vi "Swerve Math.vi"(9 "Yaw":dbl=-5.71, 10 "Rot. Point Y":dbl, 11 "Rot. Point X":dbl) -> (3 "Swerve Math Ouput":dbl[](array[numeric])=[0.0, 0.0, 0.0, 0.0, 0.0, 10.75, 16.677080080157918, 12.75])   [LabVIEW 2018]
uses:
  Drive Train Global.vi
  Robot Information/Robot Information Global.vi
  <vilib>/addons/control/pid/pid.llb/PID (DBL).vi
  <vilib>/addons/control/pid/NI_PID_pid.lvlib
panel:
  in  "PID gains":T1={"proportional gain (Kc)"=0.03, "integral time (Ti, min)"=0.0, "derivative time (Td, min)"=0.001} {"derivative time (Td, min)" format="%.3f"; "integral time (Ti, min)" format="%.3f"; "proportional gain (Kc)" format="%.3f"}
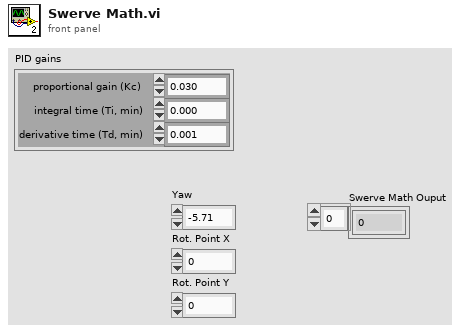
[diagram p1: front panel]
types:
  T1 = cluster{"proportional gain (Kc)":dbl, "integral time (Ti, min)":dbl, "derivative time (Td, min)":dbl}
  T2 = cluster{"Rollover":dbl, "Yaw":dbl, "Cont Yaw":dbl}
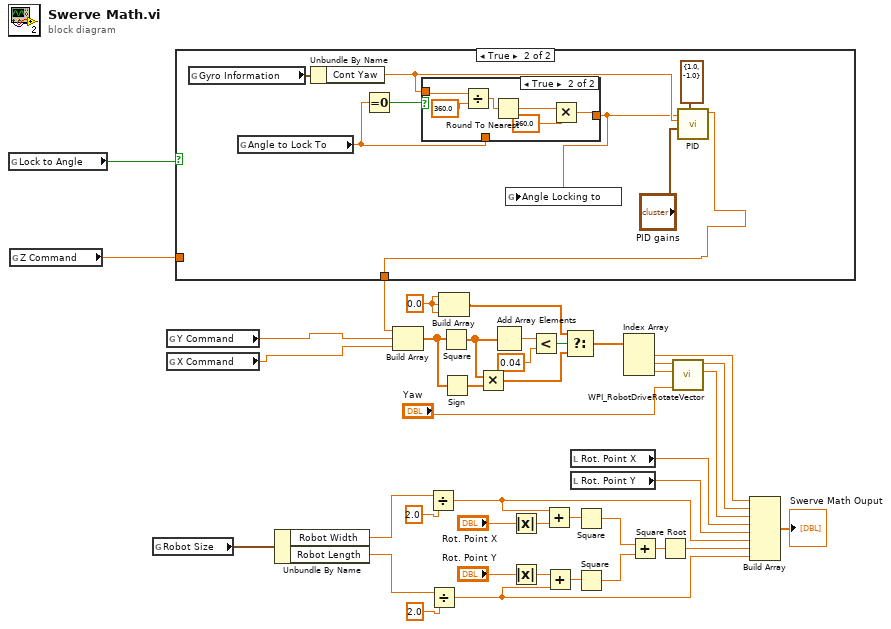
[diagram p0: block diagram]
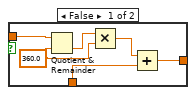
[diagram p3: hidden frame]
diagram:
  w12 = 0.0 ("element")
  n1 = global read "Drive Train Global.vi" "Lock to Angle"() -> (w4:bool)
  n2 = global read "Drive Train Global.vi" "Z Command"() -> (w5:dbl)
  n3 = global read "Robot Information Global.vi" "Robot Size"() -> (w19:cluster{"Robot Width":dbl, "Robot Length":dbl})
  n4 = global read "Drive Train Global.vi" "Y Command"() -> (w2:dbl)
  n5 = global read "Drive Train Global.vi" "X Command"() -> (w1:dbl)
  n6 = case shown="True" w4 {
    tunnel: [w42 w43] -> w3
    tunnel: w5 -> [w42 _]
    frame False {
    }
    frame True {
      n7 = global read "Drive Train Global.vi" "Gyro Information"() -> (w50:T2)
      n8 = global read "Drive Train Global.vi" "Angle to Lock To"() -> (w45:dbl)
      n9 = Unbundle By Name(w50) -> ("Cont Yaw"=w47:dbl)
      n10 = Equal To 0?(x=w45) -> (x = 0?=w44:bool)
      n11 = case shown="True" w44 {
        tunnel: w47 -> [w56 w62]
        tunnel: w45 -> [w55 _]
        tunnel: [w54 w57] -> w46
        frame False {
          w52 = 360.0 ("y")
          n12 = Quotient & Remainder(x=w56, y=w52) -> (floor(x/y)=w53:dbl)  [unwired: 1 out]
          n13 = Multiply(x=w53, y=w52) -> (x*y=w51:dbl)
          n14 = Add(x=w51, y=w55) -> (x+y=w54:dbl)
        }
        frame True {
          n15 = Divide(x=w62, y=360.0) -> (x/y=w60:dbl)
          n16 = Round To Nearest(number=w60) -> (nearest integer value=w59:dbl)
          n17 = Multiply(x=w59, y=360.0) -> (x*y=w57:dbl)
        }
      }
      n18 = global write "Drive Train Global.vi" "Angle Locking to"(w46) -> ()
      n19 = call-poly <vilib>:"PID.vi"("output range"=cluster{"output high":dbl, "output low":dbl} {"output high"=1.0, "output low"=-1.0}, "PID gains"="PID gains", "process variable"=w47, "setpoint"=w46) -> ("output"=w43:dbl)  [unwired: 6 in, 1 out]
    }
  }
  n20 = Unbundle By Name(w19) -> ("Robot Width"=w17:dbl, "Robot Length"=w18:dbl)
  n21 = Build Array(w3, w2, w1) -> (w8:dbl[])
  n22 = Divide(x=w17, y=2.0) -> (x/y=w27:dbl)
  n23 = Divide(x=w18, y=2.0) -> (x/y=w25:dbl)
  n24 = Build Array(w12, w12, w12) -> (w13:dbl[])
  n25 = Square(x=w8) -> (x^2=w10:dbl[])
  n26 = Sign(1:w8) -> (0:w11:dbl[])
  n27 = Multiply(x=w10, y=w11) -> (x*y=w9:dbl[])
  n28 = Add Array Elements(numeric array=w10) -> (sum=w16:dbl)
  n29 = Absolute Value(x="Rot. Point X") -> (abs(x)=w41:dbl)
  n30 = Absolute Value(x="Rot. Point Y") -> (abs(x)=w39:dbl)
  n31 = Less?(x=w16, y=0.04 ("x")) -> (x < y?=w14:bool)
  n32 = Add(x=w27, y=w41) -> (x+y=w40:dbl)
  n33 = Add(x=w39, y=w25) -> (x+y=w38:dbl)
  n34 = Select(t=w13, s=w14, f=w9) -> (s? t:f=w23:dbl[])
  n35 = local read "Rot. Point X"() -> (w29:dbl)
  n36 = local read "Rot. Point Y"() -> (w28:dbl)
  n37 = Square(x=w40) -> (x^2=w36:dbl)
  n38 = Square(x=w38) -> (x^2=w37:dbl)
  n39 = Index Array(array=w23) -> (element #1=w21:dbl, element #2=w24:dbl, element #3=w30:dbl)  [unwired: 3 in]
  n40 = Add(x=w36, y=w37) -> (x+y=w35:dbl)
  n41 = Square Root(x=w35) -> (sqrt(x)=w26:dbl)
  n42 = call <vilib>:"WPI_RobotDriveRotateVector.vi"("Angle"="Yaw", "X"=w30, "Y"=w24) -> ("X'"=w22:dbl, "Y'"=w20:dbl)  [unwired: 7 out]
  n43 = Build Array(w21, w20, w22, w29, w28, w27, w26, w25) -> (→"Swerve Math Ouput":dbl[])
